vi "Load.vi"(8 "error in":errorcluster, 10 "Source":string, 11 "Config from XML in":refnum<class "Config from XML.lvclass">) -> (0 "error out":errorcluster, 3 "Config from XML out":refnum<class "Config from XML.lvclass">)   [LabVIEW 2025, in "Config from XML.lvclass"]
uses:
  Config from XML.lvclass
  Config from XML.lvclass/Config from XML.ctl
  <vilib>/xml/Load XML File.vi
  <vilib>/xml/NI_XML.lvlib
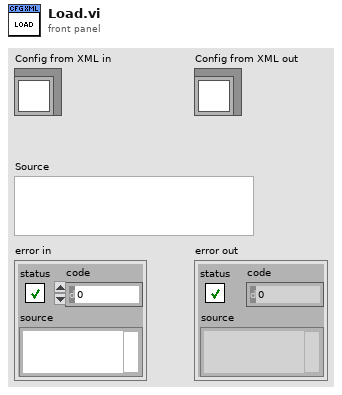
[diagram p1: front panel]
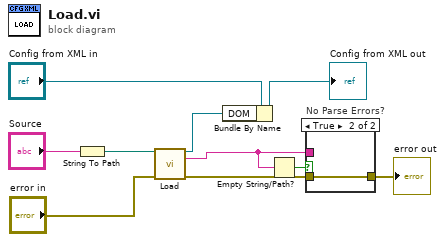
[diagram p0: block diagram]
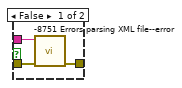
[diagram p2: hidden frame]
diagram:
  n1 = String To Path(string="Source") -> (path=w4:path)
  n2 = call-poly <vilib>:"Load.vi"("path to XML document"=w4, "error in (no error)"="error in") -> ("DOM document out"=w8:refnum<k20>, "parse errors"=w1:string, "error out"=w6:errorcluster)  [unwired: 11 in]
  n3 = Bundle By Name(cluster="Config from XML in", "DOM"=w8) -> (→"Config from XML out":refnum<class "Config from XML.lvclass">)
  n4 = Empty String/Path?(string/path=w1) -> (empty?=w2:bool)
  n5 = case "No Parse Errors?" shown="True" w2 {
    tunnel: w6 -> [w13 w14]
    tunnel: [w12 w14] -> w3
    tunnel: w1 -> [w11 _]
    frame False {
      n6 = call "-8751 Errors parsing XML file--error.vi"("error in"=w13, "Parse Errors"=w11) -> ("error out"=w12:errorcluster)  [unwired: 9 in]
    }
    frame True {
    }
  }
  "error out" <- w3
